vi "Strip Path.vi"(11 "URI in":refnum<class "URI.lvclass">) -> (2 "Stripped Segment":string, 3 "URI out":refnum<class "URI.lvclass">)   [LabVIEW 2020, in "URI.lvlib" / "URI.lvclass"]
uses:
  URI.lvclass
  URI.lvclass/URI.ctl
  URI.lvlib
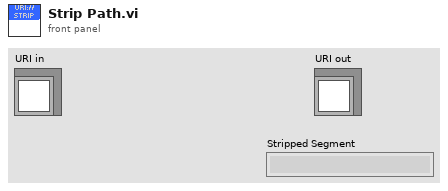
[diagram p1: front panel]
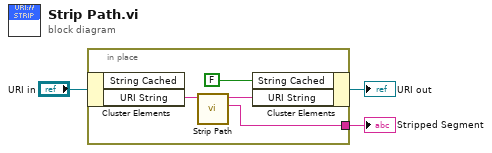
[diagram p0: block diagram]
diagram:
  n1 = in-place {
    in-place-border: [w5] -> w1
    n2 = in-place-cluster #1("URI in") -> ("URI String"=w7:string)  [unwired: 1 out]
    n3 = call "Strip Path.vi"("Path String"=w7) -> ("Stripped Segment"=w5:string, "Remaining Path"=w6:string)  [unwired: 9 in]
    n4 = in-place-cluster #1("String Cached"=FALSE, "URI String"=w6) -> (→"URI out":refnum<class "URI.lvclass">)
  }
  "Stripped Segment" <- w1
